vi "Transfered Enthalphy Evaporator Pure Water.vi"(1 "Temp Evap Water OUT":dbl[unit], 2 "Temp Evap Water IN":dbl[unit]) -> (0 "Transfered Enthalphy Evaporator (Pure) Water":dbl[unit])   [LabVIEW 2018]
panel:
  out "Enthalphy Evaporator Pure Water OUT":dbl[unit]
  out "Enthalphy Evaporator Pure Water IN":dbl[unit]
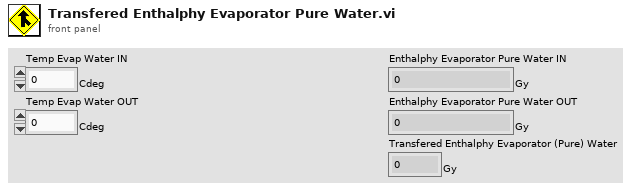
[diagram p1: front panel]
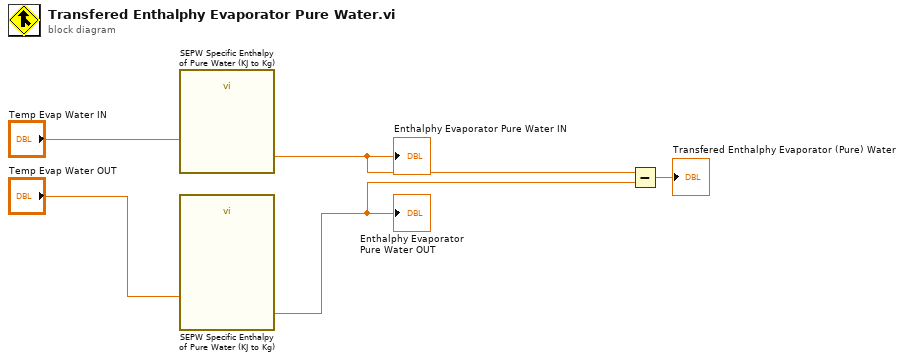
[diagram p0: block diagram]
diagram:
  n1 = call "SEPW Specific Enthalpy of Pure Water (KJ to Kg).vi"("Temp Pure Wate"="Temp Evap Water IN") -> ("SEPW"=w3:dbl[unit])
  "Enthalphy Evaporator Pure Water IN" <- w3
  n2 = call "SEPW Specific Enthalpy of Pure Water (KJ to Kg).vi"("Temp Pure Wate"="Temp Evap Water OUT") -> ("SEPW"=w2:dbl[unit])
  "Enthalphy Evaporator Pure Water OUT" <- w2
  n3 = Subtract(x=w3, y=w2) -> (x-y=→"Transfered Enthalphy Evaporator (Pure) Water":dbl[unit])
